vi "__formURL.vi"(10 "endPoint":string, 11 "REST_Client in":refnum<class "REST_Client.lvclass">) -> (2 "URL":string, 3 "REST_Client out":refnum<class "REST_Client.lvclass">)   [LabVIEW 2020, in "REST_Client.lvclass"]
uses:
  REST_Client.lvclass
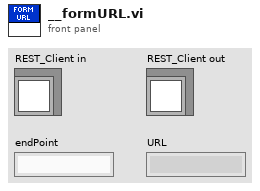
[diagram p1: front panel]
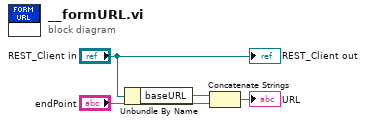
[diagram p0: block diagram]
diagram:
  n1 = Unbundle By Name("REST_Client in") -> ("baseURL"=w3:string)
  n2 = Concatenate Strings(w3, "endPoint") -> (→"URL":string)
  "REST_Client out" <- "REST_Client in"
